vi "SetVelocity.vi"(8 "error in":errorcluster, 9 "Velocity":dbl, 10 "Axial #":i32, 11 "VISA resource":refnum<visa-resource-name>) -> (0 "error out":errorcluster)   [LabVIEW 2012, in "ESP300.lvlib"]
uses:
  ESP300.lvlib
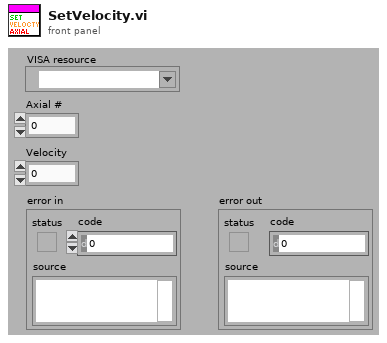
[diagram p1: front panel]
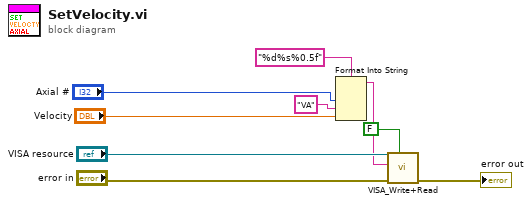
[diagram p0: block diagram]
diagram:
  n1 = Format Into String(format string="%d%s%0.5f", "Axial #", "VA" ("input 2"), "Velocity") -> (resulting string=w2:string)  [unwired: 2 in, 1 out]
  n2 = call "VISA_Write+Read.vi"("Read?(T)"=FALSE ("Read?"), "error in (no error)"="error in", "Write Buffer"=w2, "VISA resource name"="VISA resource") -> ("error out"=→"error out":errorcluster)  [unwired: 5 in, 2 out]
